vi "ballStoppers.vi"(8 "error in (no error)":errorcluster, 10 "stopperValue":dbl, 11 "stopper1 or stopper0":string="My Servo RefNum") -> (0 "error out":errorcluster)   [LabVIEW 2016]
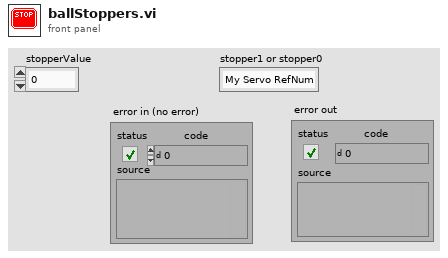
[diagram p1: front panel]
types:
  T1 = typedef "WPI_ServoDeviceRef.ctl" = cluster{"DeviceStatus":errorcluster, "PWM Channel":T2, "DeadBand":T3}
  T2 = typedef "FPGA_DIOPWMChannel.ctl" = enum8{"PWM 0", "PWM 1", "PWM 2", "PWM 3", "PWM 4", "PWM 5", "PWM 6", "PWM 7", "PWM 8", "PWM 9", "PWM MXP 0", "PWM MXP 1", "PWM MXP 2", "PWM MXP 3", "PWM MXP 4", "PWM MXP 5", "PWM MXP 6", "PWM MXP 7", "PWM MXP 8", "PWM MXP 9", "Invalid"}
  T3 = typedef "WPI_PWMDeadband.ctl" = cluster{"Name":string, "maxPositivePwm":i32, "minPositivePwm":i32, "centerPwm":i32, "maxNegativePwm":i32, "minNegativePwm":i32, "angularRange":u16}
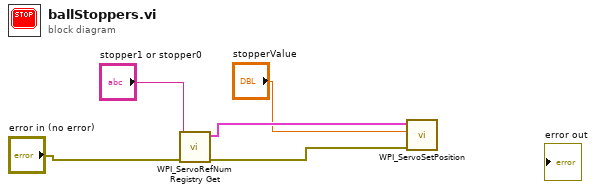
[diagram p0: block diagram]
diagram:
  n1 = call <vilib>:"WPI_ServoRefNum Registry Get.vi"("error in (no error)"="error in (no error)", "refnum name"="stopper1 or stopper0") -> ("error out"=w3:errorcluster, "ServoDeviceRef"=w4:T1)  [unwired: 8 in]
  n2 = call <vilib>:"WPI_ServoSetPosition.vi"("error in (no error)"=w3, "Position"="stopperValue", "ServoDeviceRef"=w4) -> ()  [unwired: 7 in, 2 out]
